vi "fittingParams.vi"(6 "read/write":T3, 8 "error in (no error)":errorcluster, 9 "Coagulant":T4={"flocculator volume (L)"=100.0, "clarifier volume (L)"=0.0, "dose updates per HRT"=0, "target clarified turbidity (NTU)"=0.3, "Coagulant mode"=enum."manual", "Coag dose [mg/L]"=0.0, "pump mL/rev"=0.0, "clarifier flow [L/s]"=0.5, "min Coag dose [mg/L]"=0.0, "max Coag dose [mg/L]"=0.0, "Steps"=3, "HRT response delay"=1, "Ku*"=1.0} {"HRT response delay" min=1 max=10 step=1; "Steps" min=3 step=1; "clarifier flow [L/s]" min=0.0001 max=1.0 step=0.0001; "target clarified turbidity (NTU)" min=0.1 max=5.0 step=0.01; "dose updates per HRT" min=1 max=100 step=1}, 10 "averaged data":T2) -> (0 "error out":errorcluster, 3 "Fitting Params":cluster{dbl[], "Best Linear Fit":dbl[]}[](graph), 5 "coag model":T1)   [LabVIEW 2015]
uses:
  Sensor buffer command.ctl
  coagbuffer.ctl
  calcDoseorGetGraph.ctl
  data cluster.ctl
  model type.ctl
  coag.ctl
panel:
  # "min"
  # "max"
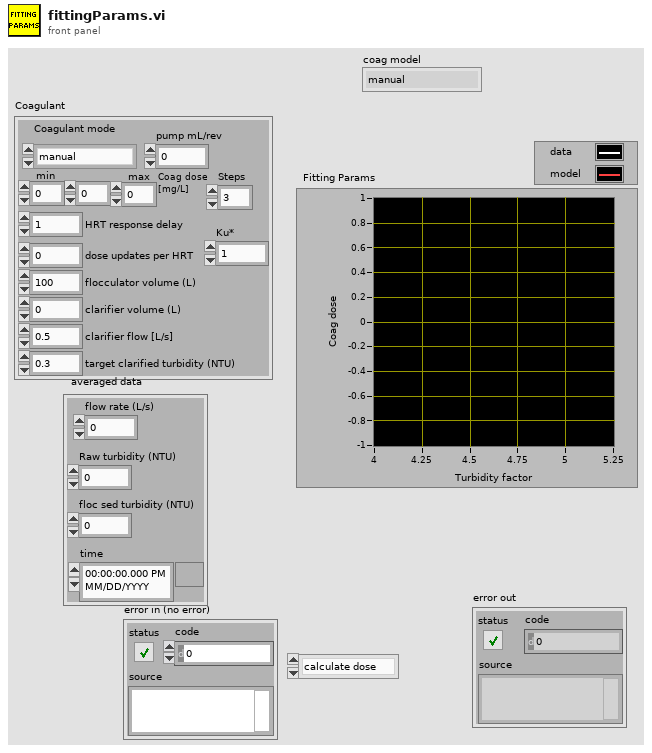
[diagram p1: front panel]
types:
  T1 = typedef "model type.ctl" = enum16{"manual", "ramp", "simple corrector", "linear regression"}
  T2 = typedef "data cluster.ctl" = cluster{"floc sed turbidity (NTU)":dbl, "Raw turbidity (NTU)":dbl, "flow rate (L/s)":dbl, "time":timestamp}
  T3 = typedef "calcDoseorGetGraph.ctl" = enum16{"calculate dose", "read graph"}
  T4 = typedef "coag.ctl" = cluster{"flocculator volume (L)":dbl, "clarifier volume (L)":dbl, "dose updates per HRT":u16, "target clarified turbidity (NTU)":dbl, "Coagulant mode":T1, "Coag dose [mg/L]":dbl, "pump mL/rev":dbl, "clarifier flow [L/s]":dbl, "min Coag dose [mg/L]":dbl, "max Coag dose [mg/L]":dbl, "Steps":u16, "HRT response delay":u32, "Ku*":dbl}
  T5 = typedef "coagbuffer.ctl" = enum16{"set buffer size", "write", "refill buffer", "read recent", "read all", "clear", "overwrite"}
  T6 = typedef "Sensor buffer command.ctl" = enum16{"set buffer size", "write", "refill buffer", "read recent", "read all", "clear"}
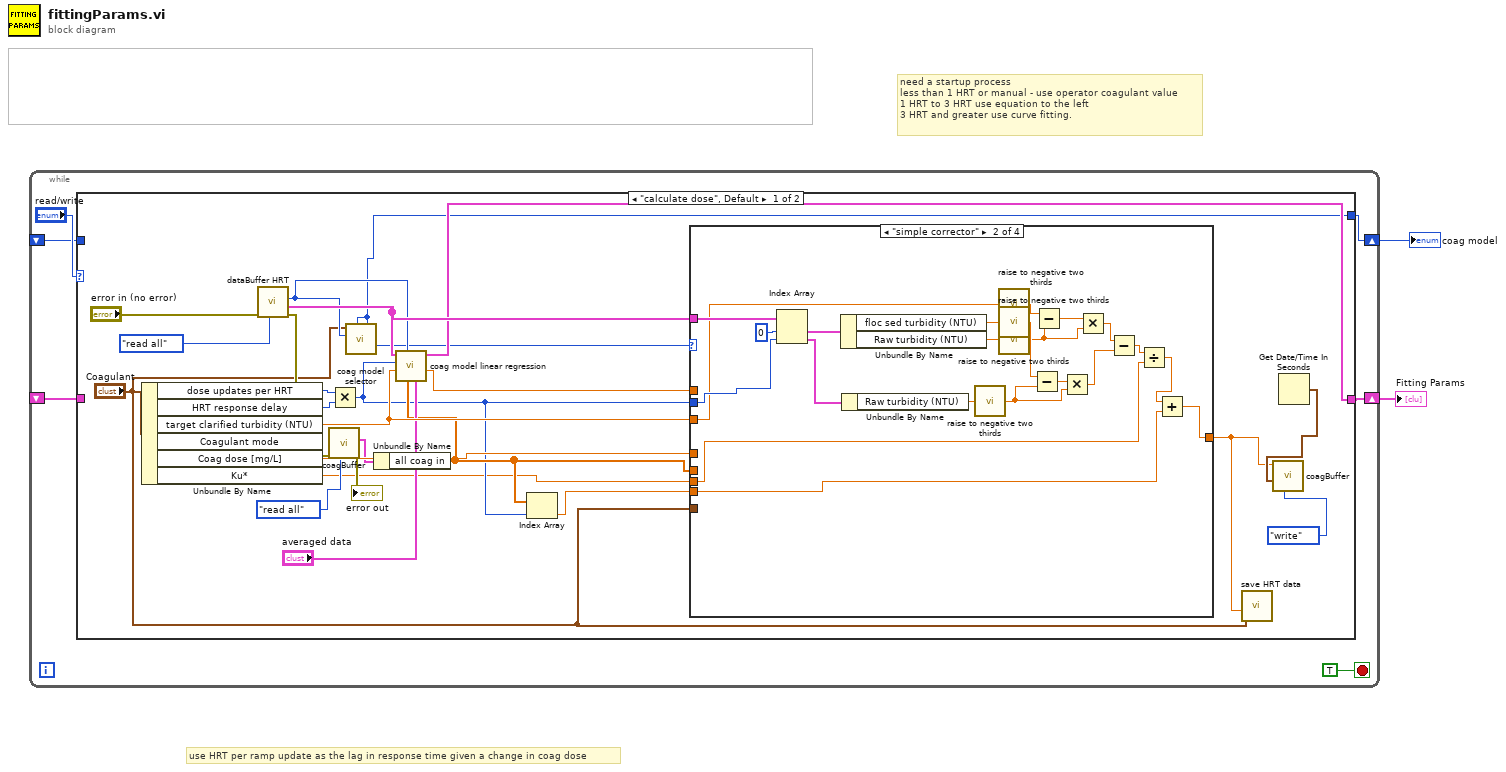
[diagram p0: block diagram]
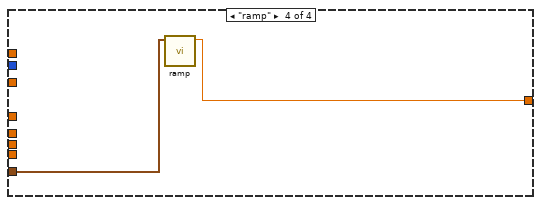
[diagram p4: hidden frame]
diagram:
  # "use HRT per ramp update as the lag in response time given a change in coag dose"
  # "need a startup process \nless than 1 HRT or manual - use operator coagulant value\n1 HRT to 3 HRT use equation to the left\n3 HRT and greater use curve fitting."
  n1 = while {
    shift-right: [w8] -> w2
    shift-left: _ -> [w7]
    shift-right: [w4] -> w1
    shift-left: _ -> [w3]
    stop <- TRUE stop-if-true
    n2 = case shown="\"calculate dose\", Default" "read/write" {
      tunnel: [w21 w60] -> w8
      tunnel: w7 -> [_ w60]
      tunnel: [w18 w59] -> w4
      tunnel: w3 -> [_ w59]
      frame "calculate dose", Default {
        n3 = Unbundle By Name("Coagulant") -> ("dose updates per HRT"=w12:u16, "HRT response delay"=w11:u32, "target clarified turbidity (NTU)"=w24:dbl, "Coag dose [mg/L]"=w28:dbl, "Ku*"=w9:dbl)  [unwired: 1 out]
        n4 = call "dataBuffer HRT.vi"("command"=Sensor_buffer_command."read all", "error in (no error)"="error in (no error)") -> ("error out"=w30:errorcluster, "all data out"=w25:T2[], "scans"=w23:i32)  [unwired: 6 in, 1 out]
        n5 = call "coagBuffer.vi"("command"=coagbuffer."read all", "error in (no error)"=w30) -> ("error out"=→"error out":errorcluster, "all data out"=w19:cluster{"time":timestamp[], "all coag in":dbl[]})  [unwired: 7 in, 1 out]
        n6 = Multiply(x=w12, y=w11) -> (x*y=w10:u32)
        n7 = call "coag model selector.vi"("scans"=w23, "Coagulant"="Coagulant") -> ("coag model"=w18:T1)  [unwired: 9 in]
        n8 = Unbundle By Name(w19) -> ("all coag in"=w15:dbl[])
        n9 = call "coag model linear regression.vi"("averaged data"="averaged data", "all coag in"=w15, "scans"=w23, "target clarified turbidity (NTU)"=w24, "dose updates per HRT"=w10, "all data in"=w25) -> ("coag dose"=w22:dbl, "Graph"=w21:cluster{dbl[], "Best Linear Fit":dbl[]}[])  [unwired: 2 in, 2 out]
        n10 = Index Array(array=w15, index=w10) -> (element=w14:dbl)
        n11 = case shown="\"simple corrector\"" w18 {
          tunnel: w25 -> [_ w55 _ _]
          tunnel: w10 -> [_ w51 _ _]
          tunnel: w15 -> [_ _ _ _]
          tunnel: w24 -> [_ w47 _ _]
          tunnel: [w33 w34 w56 w57] -> w13
          tunnel: w28 -> [w33 _ _ _]
          tunnel: w22 -> [_ _ w56 _]
          tunnel: "Coagulant" -> [_ _ _ w58]
          tunnel: w14 -> [_ w35 _ _]
          tunnel: w9 -> [_ w37 _ _]
          frame "manual", Default {
          }
          frame "simple corrector" {
            n12 = Index Array(array=w55, index #1=0 ("index"), index #2=w51) -> (element #1=w53:T2, element #2=w52:T2)
            n13 = Unbundle By Name(w53) -> ("floc sed turbidity (NTU)"=w50:dbl, "Raw turbidity (NTU)"=w49:dbl)
            n14 = Unbundle By Name(w52) -> ("Raw turbidity (NTU)"=w48:dbl)
            n15 = call "raise to negative two thirds.vi"("Numeric in"=w48) -> ("Numeric out"=w41:dbl)  [unwired: 4 in]
            n16 = call "raise to negative two thirds.vi"("Numeric in"=w47) -> ("Numeric out"=w46:dbl)  [unwired: 4 in]
            n17 = call "raise to negative two thirds.vi"("Numeric in"=w50) -> ("Numeric out"=w45:dbl)  [unwired: 4 in]
            n18 = call "raise to negative two thirds.vi"("Numeric in"=w49) -> ("Numeric out"=w43:dbl)  [unwired: 4 in]
            n19 = Subtract(x=w45, y=w41) -> (x-y=w42:dbl)
            n20 = Subtract(x=w46, y=w43) -> (x-y=w44:dbl)
            n21 = Multiply(x=w42, y=w41) -> (x*y=w39:dbl)
            n22 = Multiply(x=w44, y=w43) -> (x*y=w40:dbl)
            n23 = Subtract(x=w40, y=w39) -> (x-y=w38:dbl)
            n24 = Divide(x=w38, y=w37) -> (x/y=w36:dbl)
            n25 = Add(x=w36, y=w35) -> (x+y=w34:dbl)
          }
          frame "linear regression" {
          }
          frame "ramp" {
            n26 = call "ramp.vi"("Coagulant"=w58) -> ("Coag dose"=w57:dbl)  [unwired: 10 in]
          }
        }
        n27 = call "save HRT data.vi"("coagulant dose"=w13, "Coagulant"="Coagulant") -> ()  [unwired: 10 in]
        n28 = Get Date/Time In Seconds() -> (seconds since 1Jan1904=w16:timestamp)
        n29 = call "coagBuffer.vi"("command"=coagbuffer."write", "Time Stamp"=w16, "Coag dose"=w13) -> ()  [unwired: 6 in, 3 out]
      }
      frame "read graph" {
      }
    }
  }
  "Fitting Params" <- w2
  "coag model" <- w1
